vi "UpdatePreviousLoadedViList.vi"(8 "error in (no error)":errorcluster, 11 "HmiSchedulerAppContextIn":T1) -> (0 "error out":errorcluster, 3 "HmiSchedulerAppContextOut":T1)   [LabVIEW 2011]
uses:
  HmiSchedulerAppConfig.ctl
  030 - EVENTS/03 - ToMessageHandlerProcess/ToMessageHandlerEvent.ctl
  030 - EVENTS/03 - ToMessageHandlerProcess/enumMessageCriticity.ctl
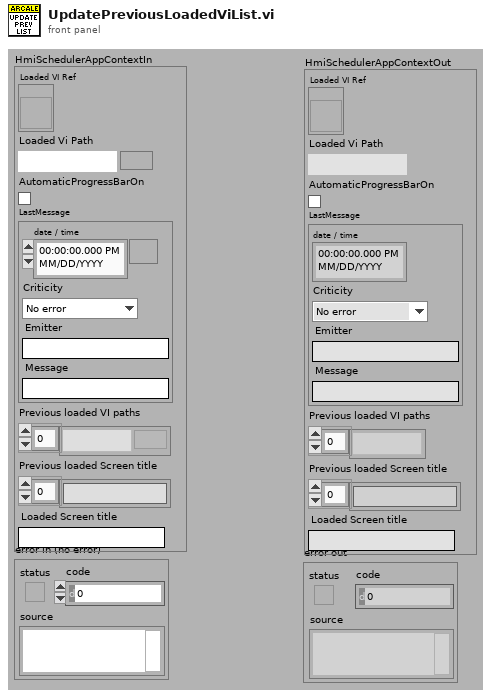
[diagram p1: front panel]
types:
  T1 = typedef "HmiSchedulerAppConfig.ctl" = cluster{"Loaded VI Ref":refnum<vi>, "Loaded Vi Path":path, "AutomaticProgressBarOn":bool, "LastMessage":T2, "Previous loaded VI paths":path[], "Previous loaded Screen title":string[], "Loaded Screen title":string}
  T2 = typedef "ToMessageHandlerEvent.ctl" = cluster{"date / time":timestamp, "Criticity":T3, "Emitter":string, "Message":string}
  T3 = typedef "enumMessageCriticity.ctl" = enum16{"No error", "Info", "Warning", "Error", "Fatal error"}
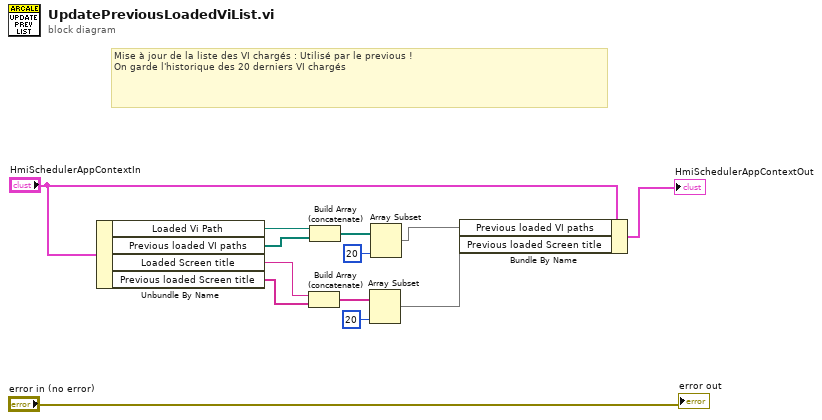
[diagram p0: block diagram]
diagram:
  # "Mise à jour de la liste des VI chargés : Utilisé par le previous !\nOn garde l'historique des 20 derniers VI chargés"
  n1 = Unbundle By Name("HmiSchedulerAppContextIn") -> ("Loaded Vi Path"=w11:path, "Previous loaded VI paths"=w10:path[], "Loaded Screen title"=w4:string, "Previous loaded Screen title"=w3:string[])
  n2 = Build Array (concatenate)(w4, w3) -> (w5:string[])
  n3 = Build Array (concatenate)(w11, w10) -> (w9:path[])
  n4 = Array Subset(array=w5, length=20) -> (w2:string[])  [unwired: 1 in]
  n5 = Array Subset(array=w9, length=20) -> (w8:path[])  [unwired: 1 in]
  n6 = Bundle By Name(cluster="HmiSchedulerAppContextIn", "Previous loaded VI paths"=w8, "Previous loaded Screen title"=w2) -> (→"HmiSchedulerAppContextOut":T1)
  "error out" <- "error in (no error)"
